vi "sub_Demod_Frame.vi"(5 "Packet Length [samples]":i32, 6 "matched filter coefficients":dbl[](array[numeric]) format="%^.2e", 7 "Expected Xcorr Index":i32, 8 "Packet Parameters in":T2={"Length of sync sequence (50)"=50, "Number of message bits"=128, "Number of guardbits"=40, "Sync PN sequence order (31)"=31, "Number of header bits"=16, "Packet Pad [samples]"=0}, 9 "PSK system parameters":T1, 10 "Sync Sequence Waveform":cdb[](array[numeric]), 11 "Input Complex Waveform":T3={"t0"=0.0, "dt"=1.0, "Y"=[]} {"Y" format="%.3f"; "dt" format="%^.2e"; "t0" format="%.4f"}) -> (1 "Max Xcorr Index":i32, 2 "output bit stream":i8[](array[numeric]), 3 "Xcorr Waveform":cdb[](array[numeric]))   [LabVIEW 2014]
uses:
  <vilib>/addons/Modulation/Analog/controls/Complex Data Waveform.ctl
  <vilib>/addons/Modulation/Digital/General/MT Apply Matched Filter (Generic).vi
  <vilib>/addons/Modulation/Digital/General/MT Map PSK Symbols to Bits.vi
  <vilib>/addons/Modulation/niDMT.lvlib
  <vilib>/addons/Modulation/niAMT.lvlib
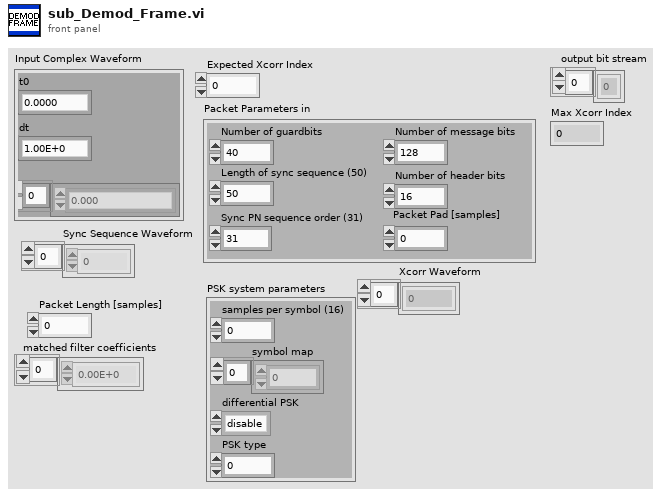
[diagram p1: front panel]
types:
  T1 = cluster{"samples per symbol (16)":i32, "symbol map":cdb[], "differential PSK":enum16{"disable", "enable"}, "PSK type":u16}
  T2 = cluster{"Length of sync sequence (50)":i32, "Number of message bits":i32, "Number of guardbits":i32, "Sync PN sequence order (31)":i32, "Number of header bits":i32, "Packet Pad [samples]":i32}
  T3 = typedef "niAMT.lvlib/Complex Data Waveform.ctl" = cluster{"t0":dbl, "dt":dbl, "Y":cdb[]}
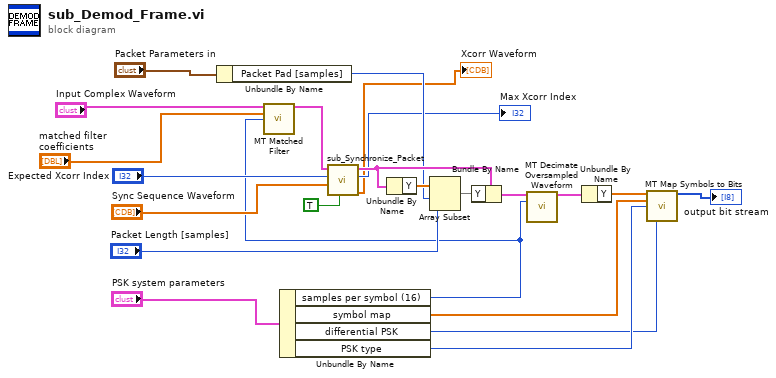
[diagram p0: block diagram]
diagram:
  n1 = Unbundle By Name("Packet Parameters in") -> ("Packet Pad [samples]"=w12:i32)
  n2 = Unbundle By Name("PSK system parameters") -> ("samples per symbol (16)"=w3:i32, "symbol map"=w10:cdb[], "differential PSK"=w8:enum16{"disable", "enable"}, "PSK type"=w9:u16)
  n3 = call-poly <vilib>:"MT Matched Filter.vi"("input complex waveform"="Input Complex Waveform", "matched filter coefficients"="matched filter coefficients", "samples per symbol (16)"=w3) -> ("output complex waveform"=w6:T3)  [unwired: 11 in, 1 out]
  n4 = call "sub_Synchronize_Packet.vi"("Realign Waveform (T)"=TRUE, "Sync Sequence Waveform"="Sync Sequence Waveform", "Expected Sync Index"="Expected Xcorr Index", "Input Complex Waveform"=w6) -> ("Xcorr Waveform"=→"Xcorr Waveform":cdb[], "Max Xcorr Index"=→"Max Xcorr Index":i32, "Output Complex Waveform"=w21:T3)  [unwired: 4 in, 1 out]
  n5 = Unbundle By Name(w21) -> ("Y"=w22:cdb[])
  n6 = Array Subset(array=w22, index=w12, length="Packet Length [samples]") -> (w23:cdb[])
  n7 = Bundle By Name(cluster=w21, "Y"=w23) -> (w20:T3)
  n8 = call <vilib>:"MT Decimate Oversampled Waveform.vi"("input complex waveform"=w20, "decimation factor"=w3) -> ("output complex waveform"=w18:T3)  [unwired: 12 in, 1 out]
  n9 = Unbundle By Name(w18) -> ("Y"=w19:cdb[])
  n10 = call-poly <vilib>:"MT Map Symbols to Bits.vi"("symbols"=w19, "symbol map"=w10, "PSK type"=w9, "differential PSK"=w8) -> ("output bit stream"=→"output bit stream":i8[])  [unwired: 10 in, 1 out]
